vi "Untitled 6 (SubVI).vi"(6 "core width\n   (mrad)":dbl, 7 "sigma (mrad) in":dbl, 9 "Numeric 7":i32, 10 "Fermi angle\n   (mrad)":dbl, 11 "Numeric 6":i32) -> (1 "Numeric 3":dbl, 2 "Numeric 2":dbl, 3 "Numeric 5":i32, 4 "Numeric 4":dbl, 5 "Numeric":dbl)   [LabVIEW 2013]
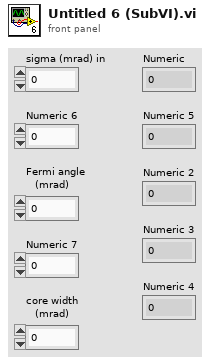
[diagram p1: front panel]
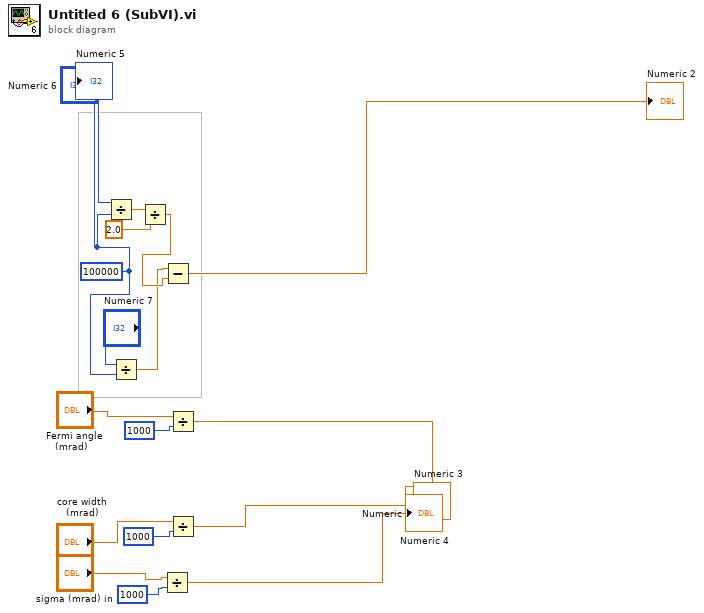
[diagram p0: block diagram]
diagram:
  w11 = 100000
  n1 = Divide(x="Numeric 6", y=w11) -> (x/y=w3:dbl)
  n2 = Divide(x="Numeric 7", y=w11) -> (x/y=w1:dbl)
  n3 = Divide(x=w3, y=2.0) -> (x/y=w5:dbl)
  n4 = Divide(x="sigma (mrad) in", y=1000) -> (x/y=→"Numeric":dbl)
  n5 = Subtract(x=w1, y=w5) -> (x-y=→"Numeric 2":dbl)
  n6 = Divide(x="Fermi angle\n   (mrad)", y=1000) -> (x/y=→"Numeric 3":dbl)
  n7 = Divide(x="core width\n   (mrad)", y=1000) -> (x/y=→"Numeric 4":dbl)
  "Numeric 5" <- w11
